vi "toast.vi"(8 "error in (no error)":errorcluster, 11 "ToasterOven in":refnum<class "ToasterOven.lvclass">) -> (0 "error out":errorcluster, 3 "ToasterOven out":refnum<class "ToasterOven.lvclass">)   [LabVIEW 2010, in "ToasterOven.lvclass"]
uses:
  ToasterOven.lvclass
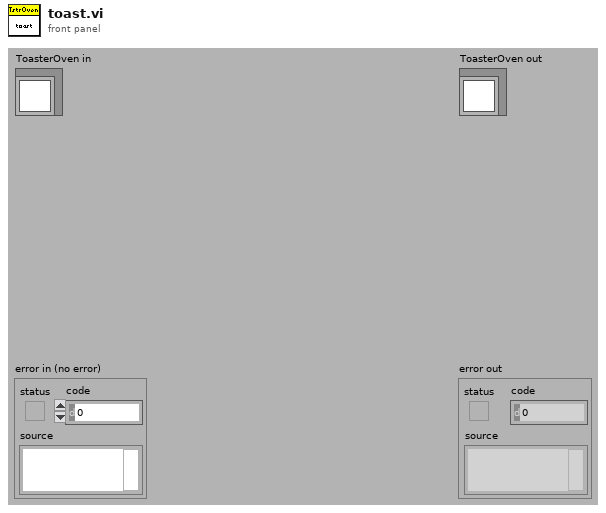
[diagram p1: front panel]
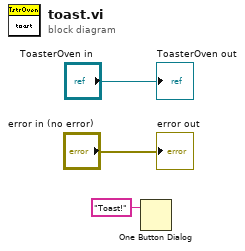
[diagram p0: block diagram]
diagram:
  n1 = One Button Dialog(message="Toast!") -> ()  [unwired: 1 in, 1 out]
  "error out" <- "error in (no error)"
  "ToasterOven out" <- "ToasterOven in"
